vi "BLE_GetRandNumber.vi"(0 "ServicesUUIDs Value":string[][](array[string]), 5 "UUID L1L2L3":string, 9 "UUID Author":string, 11 "error in (no error)":errorcluster) -> (4 "RNDnumber":u8[](array[numeric]) format="%.0x", 6 "Found?":bool, 15 "error out":errorcluster)   [LabVIEW 2020]
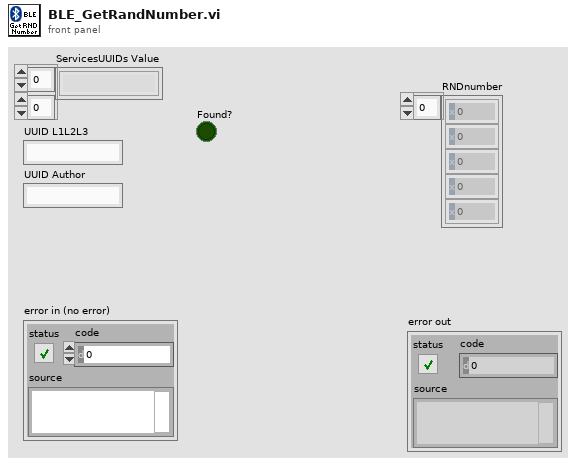
[diagram p1: front panel]
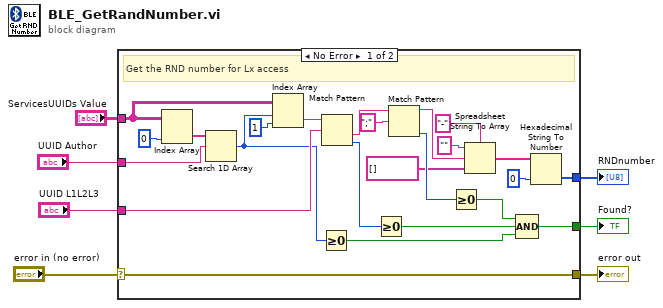
[diagram p0: block diagram]
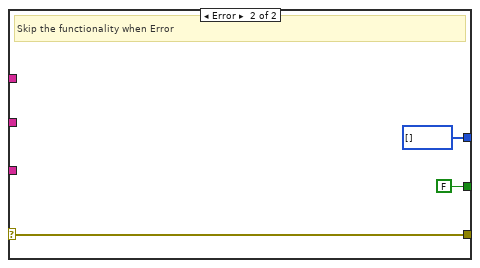
[diagram p2: hidden frame]
diagram:
  n1 = case shown="No Error" "error in (no error)" {
    selector: "error in (no error)" -> [w8 w34]
    tunnel: "UUID L1L2L3" -> [w28 _]
    tunnel: "ServicesUUIDs Value" -> [w25 _]
    tunnel: "UUID Author" -> [w24 _]
    tunnel: [w16 FALSE] -> w4
    tunnel: [w10 u8[] []] -> w3
    tunnel: [w8 w34] -> w2
    frame No Error {
      # "Get the RND number for Lx access"
      n2 = Index Array(array=w25, index (col)=0 ("index (row)")) -> (element=w23:string[])  [unwired: 1 in]
      n3 = Search 1D Array(1D array=w23, element=w24) -> (index of element=w22:i32)  [unwired: 1 in]
      n4 = Index Array(array=w25, index (row)=w22, index (col)=1 ("disabled index (col)")) -> (element=w27:string)
      n5 = Greater Or Equal To 0?(x=w22) -> (x >= 0?=w17:bool)
      n6 = Match Pattern(string=w27, regular expression=w28) -> (after substring=w29:string, offset past match=w21:i32)  [unwired: 1 in, 2 out]
      n7 = Greater Or Equal To 0?(x=w21) -> (x >= 0?=w18:bool)
      n8 = Match Pattern(string=w29, regular expression=";") -> (before substring=w15:string, offset past match=w20:i32)  [unwired: 1 in, 2 out]
      n9 = Greater Or Equal To 0?(x=w20) -> (x >= 0?=w19:bool)
      n10 = Spreadsheet String To Array(delimiter (Tab)="-", format string="", spreadsheet string=w15, array type (2D Dbl)=string[] []) -> (array=w11:string[])
      n11 = Compound Arithmetic op=AND(w19, w18, w17) -> (w16:bool)
      n12 = Hexadecimal String To Number(string=w11, default (0uL)=u8 0 ("default (0 U32)")) -> (number=w10:u8[])  [unwired: 1 in, 1 out]
    }
    frame Error {
      # "Skip the functionality when Error"
    }
  }
  "Found?" <- w4
  "RNDnumber" <- w3
  "error out" <- w2
